vi "2_VNA_smith_reflection_(Smith_main_TH).vi"() -> ()   [LabVIEW 2013]
uses:
  support_functions/_VNA_smith_reflection_GLOBALVARIABLES.vi
panel:
  in  "Yokogawa Address":refnum<visa-resource-name>="GPIB0::25::INSTR"
  in  "Background?":bool
  in  "Tab Control":enum32{"Page 1"}(tab)
  in  "Save?":bool=TRUE
  in  "Name":string="data_labView_Mar'18_"
  out "Normalised amplitude":cluster{dbl[], dbl[]}[](graph)
  in  "Smoothing points":i32
  in  "Boolean":bool=TRUE
  out "Amplitude Background":cluster{dbl[], dbl[]}[](graph)
  out "Amplitude":cluster{dbl[], dbl[]}[](graph)
  in  "?":enum32{"VNA"}(tab)
  in  "Center Freq (Hz)":dbl=6953330000.0 caption="Center Freq (Hz):" format="%#.6p"
  in  "Span Freq:":dbl=50000000.0 caption="Span Freq (Hz)" format="%#.3p"
  in  "Points:":i32=201 caption="Points"
  in  "Bandwidth (Hz)":dbl[](array[numeric])=[3.0, 3.0, 3.0, 5.0, 5.0, 5.0, 5.0]
  in  "VNA Power (dBm)":dbl[](array[numeric])=[-50.0, -45.0, -40.0, -35.0, -30.0, -25.0, -20.0]
  in  "I resonance (mA)":dbl step=2e-05
  in  "I background (mA)":dbl step=2e-05
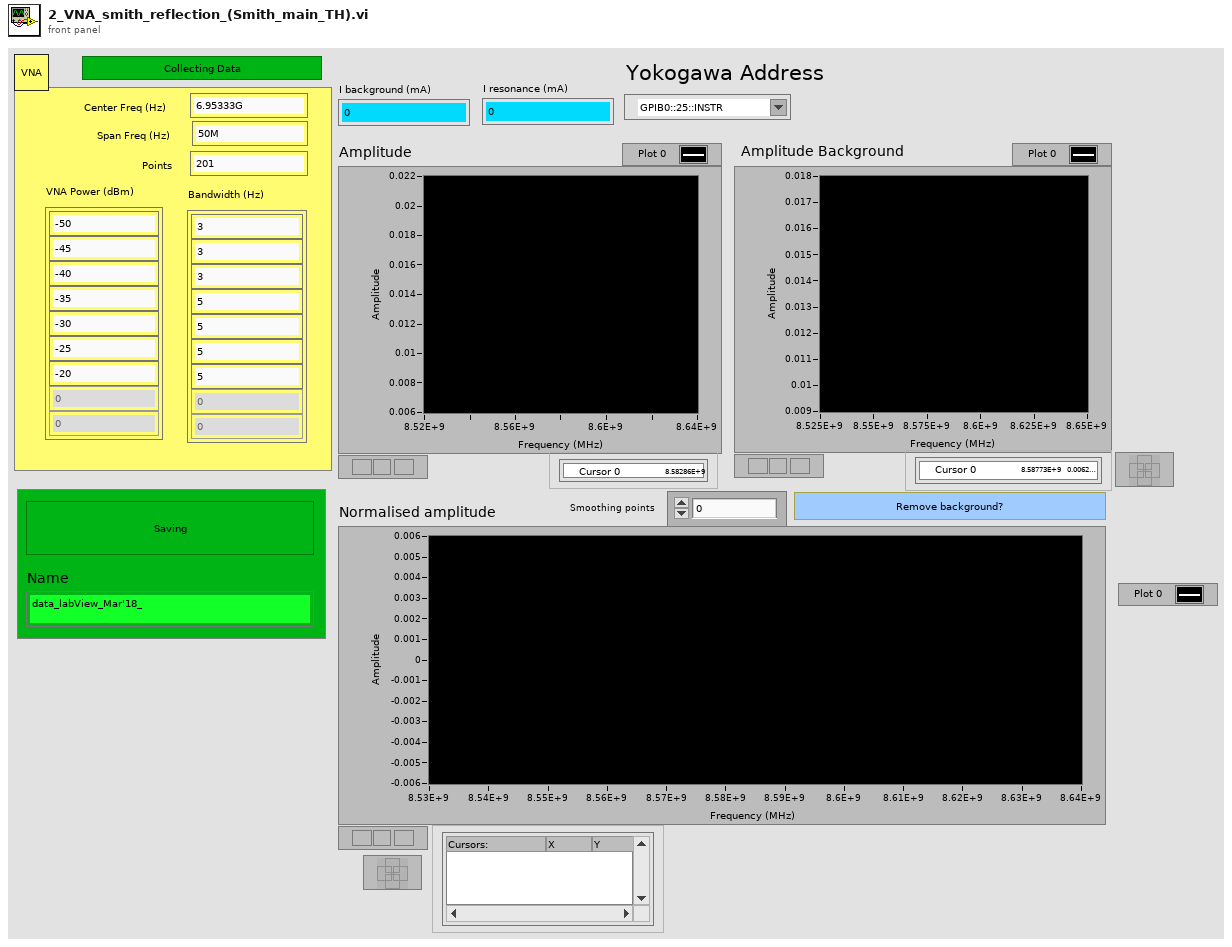
[diagram p1: front panel]
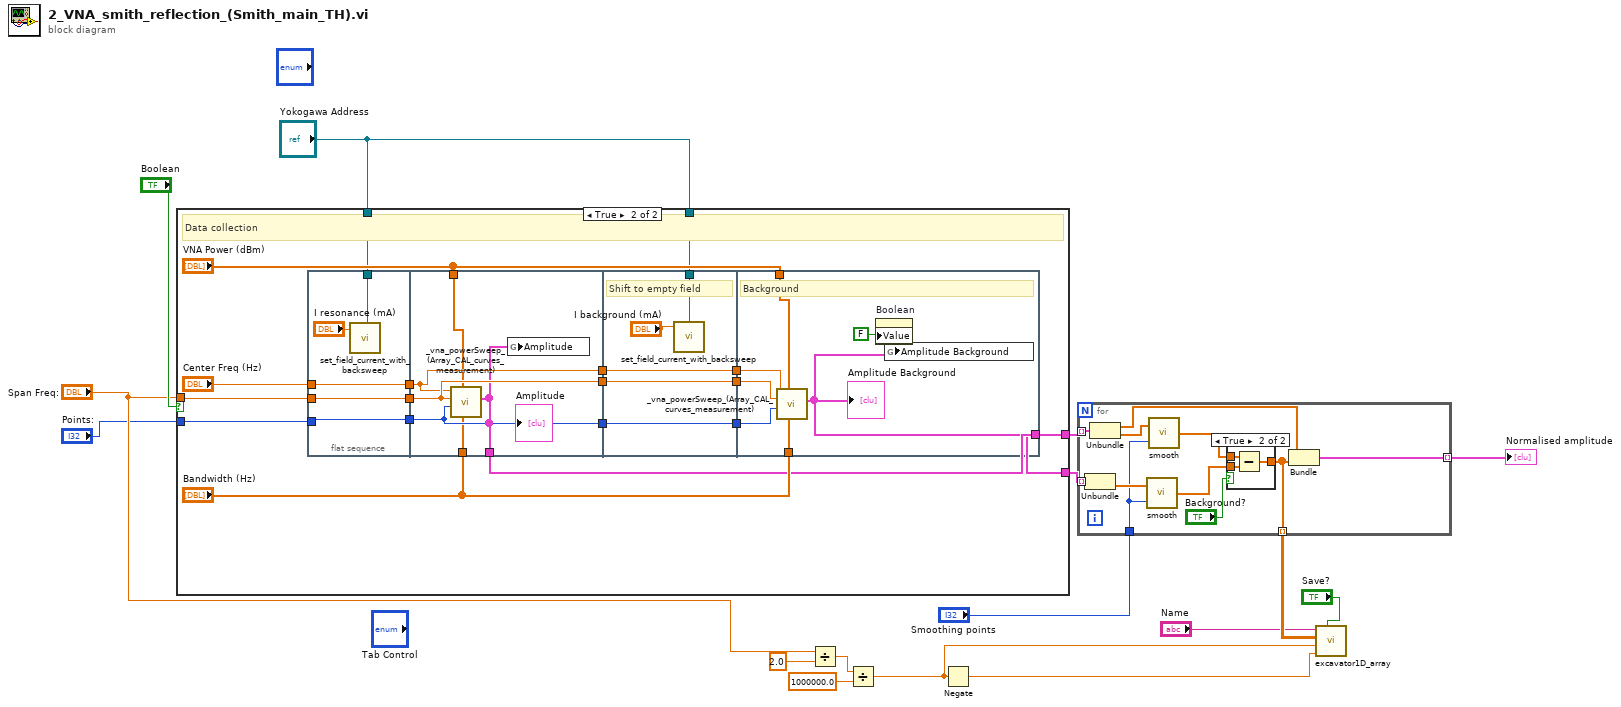
[diagram p0: block diagram]
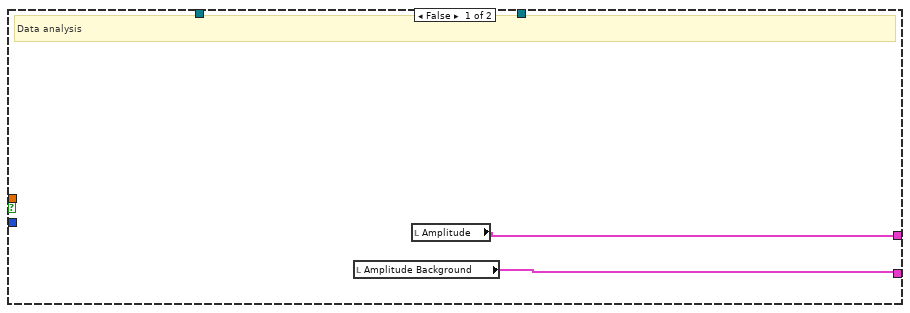
[diagram p3: hidden frame]
diagram:
  n1 = case shown="True" "Boolean" {
    tunnel: [w18 w20] -> w13
    tunnel: [w17 w19] -> w14
    tunnel: "Span Freq:" -> [_ w25]
    tunnel: "Yokogawa Address" -> [_ w23]
    tunnel: "Yokogawa Address" -> [_ w22]
    tunnel: "Points:" -> [_ w21]
    frame False {
      # "Data analysis"
      n2 = local read "Amplitude Background"() -> (w17:cluster{dbl[], dbl[]}[])
      n3 = local read "Amplitude"() -> (w18:cluster{dbl[], dbl[]}[])
    }
    frame True {
      # "Data collection"
      n4 = flat-sequence {
        tunnel: w25 -> [w40]
        tunnel: [w40] -> w36
        tunnel: [w39] -> w35
        tunnel: "Center Freq (Hz)" -> [w39]
        tunnel: [w38] -> w34
        tunnel: w21 -> [w38]
        tunnel: w23 -> [w37]
        tunnel: w36 -> [w47]
        tunnel: [w47] -> w33
        tunnel: w35 -> [w46]
        tunnel: [w46] -> w32
        tunnel: w34 -> [w45]
        tunnel: [w45] -> w31
        tunnel: "Bandwidth (Hz)" -> [w44]
        tunnel: "VNA Power (dBm)" -> [w43]
        tunnel: [w42] -> w20
        tunnel: [w51] -> w30
        tunnel: w33 -> [w51]
        tunnel: [w50] -> w29
        tunnel: w32 -> [w50]
        tunnel: [w49] -> w28
        tunnel: w31 -> [w49]
        tunnel: w22 -> [w48]
        tunnel: w30 -> [w59]
        tunnel: w29 -> [w58]
        tunnel: w28 -> [w57]
        tunnel: "Bandwidth (Hz)" -> [w56]
        tunnel: "VNA Power (dBm)" -> [w55]
        tunnel: [w53] -> w19
        frame #0 {
          n5 = call "set_field_current_with_backsweep.vi"("Yokogawa Address"=w37, "I mA"="I resonance (mA)") -> ()  [unwired: 3 in, 1 out]
        }
        frame #1 {
          n6 = call "_vna_powerSweep_(Array_CAL_curves_measurement).vi"("Bandwidth (Hz)"=w44, "VNA Power (dBm)"=w43, "Points:"=w45, "Span Freq:"=w47, "Center Freq (Hz)"=w46) -> ("Amplitude"=w42:cluster{dbl[], dbl[]}[])  [unwired: 1 in, 3 out]
          "Amplitude" <- w42
          n7 = global write "_VNA_smith_reflection_GLOBALVARIABLES.vi" "Amplitude"(w42) -> ()
        }
        frame #2 {
          # "Shift to empty field"
          n8 = call "set_field_current_with_backsweep.vi"("Yokogawa Address"=w48, "I mA"="I background (mA)") -> ()  [unwired: 3 in, 1 out]
        }
        frame #3 {
          # "Background"
          n9 = call "_vna_powerSweep_(Array_CAL_curves_measurement).vi"("Bandwidth (Hz)"=w56, "VNA Power (dBm)"=w55, "Points:"=w57, "Span Freq:"=w59, "Center Freq (Hz)"=w58) -> ("Amplitude"=w53:cluster{dbl[], dbl[]}[])  [unwired: 1 in, 3 out]
          "Amplitude Background" <- w53
          n10 = property on="Boolean" class="Bool (strict)"("Value"=FALSE ("Boolean")) -> ()  [unwired: 2 in, 2 out]
          n11 = global write "_VNA_smith_reflection_GLOBALVARIABLES.vi" "Amplitude Background"(w53) -> ()
        }
      }
    }
  }
  n12 = Divide(x="Span Freq:", y=2.0) -> (x/y=w7:dbl)
  n13 = Divide(x=w7, y=1000000.0) -> (x/y=w4:dbl)
  n14 = Negate(x=w4) -> (-x=w5:dbl)
  n15 = for {
    tunnel: w13 -> [w70] mode=indexing
    tunnel: "Smoothing points" -> [w67]
    tunnel: w14 -> [w68] mode=indexing
    tunnel: [w62] -> w12 mode=indexing
    tunnel: [w63] -> w11 mode=indexing
    n16 = Unbundle(w68) -> (w69:dbl[])  [unwired: 1 out]
    n17 = Unbundle(w70) -> (w65:dbl[], w66:dbl[])
    n18 = call "smooth.vi"("length"=w67, "Array in"=w69) -> ("Array out"=w60:dbl[])
    n19 = call "smooth.vi"("length"=w67, "Array in"=w66) -> ("Array out"=w61:dbl[])
    n20 = case shown="True" "Background?" {
      tunnel: w61 -> [w71 w74]
      tunnel: w60 -> [_ w73]
      tunnel: [w71 w72] -> w63
      frame False {
      }
      frame True {
        n21 = Subtract(x=w74, y=w73) -> (x-y=w72:dbl[])
      }
    }
    n22 = Bundle(w65, "Array out"=w63) -> (w62:cluster{dbl[], "Array out":dbl[]})  [unwired: 1 in]
  }
  "Normalised amplitude" <- w12
  n23 = call "excavator1D_array.vi"("Name"="Name", "Array"=w11, "x_max"=w4, "x_min"=w5, "Save?"="Save?") -> ()  [unwired: 1 out]
